vi "Create.vi"   [LabVIEW 2020, in "feature_detection.lvlib" / "QR Code Encoder.lvclass"]
doc: "Create a QR Code Generator."
uses:
  QR Code Encoder.lvclass
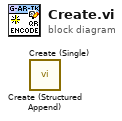
[diagram p0: block diagram]
diagram:
  n1 = call "Create (Structured Append).vi"() -> ()  [unwired: 10 in, 2 out]
  n2 = call "Create (Single).vi"() -> ()  [unwired: 10 in, 2 out]
